vi "Test I-V Pattern.vi"() -> ()   [LabVIEW 2021]
uses:
  Waform generation/I-V parameters.ctl
  Waform generation/Waveform parameters.ctl
panel:
  out "I-V waveform 2":dbl[](graph)
  in  "Full output  bit range":i32=8192 format="0x%x (%d)"
  out "min value":i16
  out "max value":i16
  out "In range?":bool
  out "Waveform parameters out":T1={"Start magnitude"=0.0, "Magnitude increment"=0.0, "Number of pulses"=0, "Ramp length"=0, "Top  length"=0, "Threshold "=3000, "Processing delay"=240, "Stop after"=1, "Detector window"=480, "Upper limit"=32767, "Lower limit"=32767} {"Lower limit" format="%d (0x%x)"; "Upper limit" format="%d (0x%x)"; "Detector window" format="%dpts"; "Stop after" format="%d sweep(s)"}
  out "DAC waveform":i16[](graph)
  in  "Input range":dbl=1.0 format="%#_6p"
  in  "I-V parameters":T2={"Start magnitude"=0.2, "Magnitude increment"=0.05, "End magnitude"=0.5, "Ramp length"=50, "Top  length"=60, "Threshold "=0.2, "Processing delay"=5, "Output gain "=0.5, "Interpolation"=64, "Stop after"=55, "Detector window"=480} {"Detector window" format="%dpts"; "Stop after" format="%d sweep(s)"; "Output gain" format="%#_6pA/V"; "Processing delay" format="%dpts"; "Threshold" format="%#_6pV"; "Top  length" format="%dpts"; "Ramp length" format="%dpts"; "End magnitude" format="%#_6pA"; "Magnitude increment" format="%#_6pA"; "Start magnitude" format="%#_6pA"}
  # "Waveform parameters"
  # "Detector parameters"
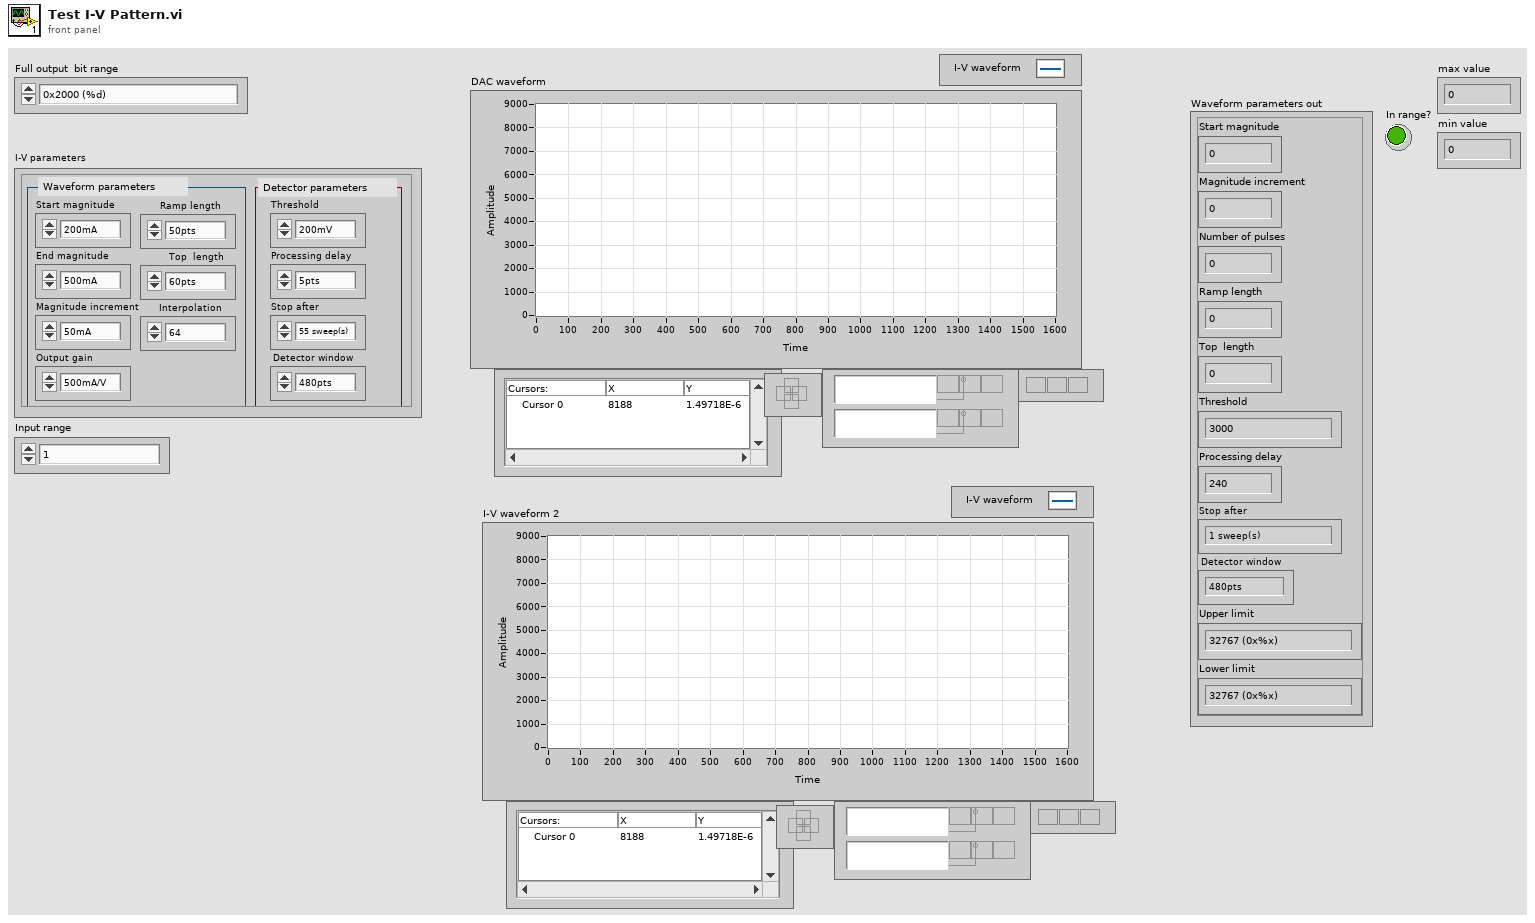
[diagram p1: front panel]
types:
  T1 = typedef "Waveform parameters.ctl" = cluster{"Start magnitude":dbl, "Magnitude increment":dbl, "Number of pulses":i32, "Ramp length":i32, "Top  length":i32, "Threshold ":i32, "Processing delay":u16, "Stop after":u16, "Detector window":i32, "Upper limit":i16, "Lower limit":i16}
  T2 = typedef "I-V parameters.ctl" = cluster{"Start magnitude":dbl, "Magnitude increment":dbl, "End magnitude":dbl, "Ramp length":i32, "Top  length":i32, "Threshold ":dbl, "Processing delay":u16, "Output gain ":dbl, "Interpolation":i32, "Stop after":u16, "Detector window":i32}
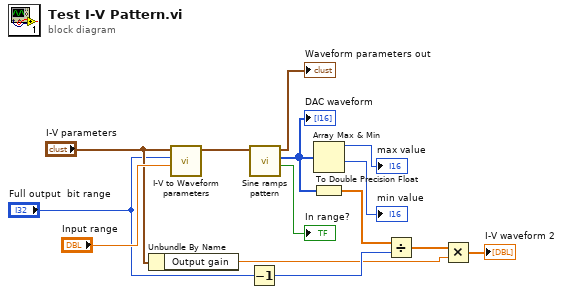
[diagram p0: block diagram]
diagram:
  n1 = Unbundle By Name("I-V parameters") -> ("Output gain"=w2:dbl)
  n2 = call "I-V to Waveform parameters.vi"("Input range"="Input range", "Full output  bit range"="Full output  bit range", "I-V parameters"="I-V parameters") -> ("Waveform parameters out"=w14:T1)  [unwired: 8 in]
  n3 = Decrement(x="Full output  bit range") -> (x-1=w4:i32)
  n4 = call "Sine ramps pattern.vi"("Waveform parameters 2"=w14) -> ("In range?"=→"In range?":bool, "Waveform"=w7:i16[], "Waveform parameters out"=→"Waveform parameters out":T1)  [unwired: 7 in]
  "DAC waveform" <- w7
  n5 = Array Max & Min(array=w7) -> (max value=→"max value":i16, min value=→"min value":i16)  [unwired: 2 out]
  n6 = To Double Precision Float(number=w7) -> (double precision float=w6:dbl[])
  n7 = Divide(x=w6, y=w4) -> (x/y=w3:dbl[])
  n8 = Multiply(x=w3, y=w2) -> (x*y=→"I-V waveform 2":dbl[])
